vi "change_array_rows.vi"(9 "Scan Parameters 3":refnum<vi>, 10 "Scan Parameters":T1={"Initial Values"=[4.0], "Final Values"=[10.0, 0.0, 0.0], "Step Sizes"=[0.5, 0.0, 0.0], "Parameters to Change"=[enum."Static Voltage", enum."Static Voltage", enum."Static Voltage"], "Channels to Change"=[1.0, 0.0, 0.0], "Number of Parameters to Scan"=1, "Parameter Nickname (no spaces)"=["drop time"], "Scan Base Name"="BlueDetuning_", "Raw_Data Folder"=path "C:/Users/Rydberg/Documents/Data/Raw_Data/84Sr/2014.12.13"} {"Number of Parameters to Scan" min=1}) -> (2 "Scan Parameters 2":refnum<vi>)   [LabVIEW 2013]
uses:
  Controls/ScanParameters/ScanParametersPanel.ctl
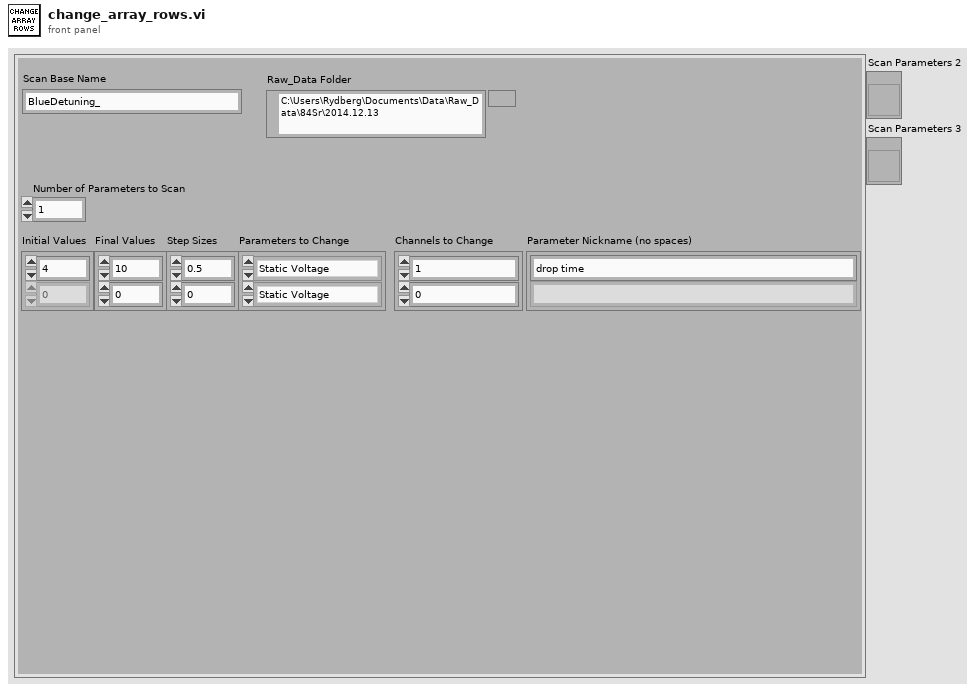
[diagram p1: front panel]
types:
  T1 = typedef "ScanParametersPanel.ctl" = cluster{"Initial Values":dbl[], "Final Values":dbl[], "Step Sizes":dbl[], "Parameters to Change":enum16{"PulseBlaster", "Static Voltage"}[], "Channels to Change":dbl[], "Number of Parameters to Scan":i32, "Parameter Nickname (no spaces)":string[], "Scan Base Name":string, "Raw_Data Folder":path}
  T2 = cluster{"Initial Values":refnum<vi>, "Final Values":refnum<vi>, "Step Sizes":refnum<vi>, "Channels to Change":refnum<vi>}
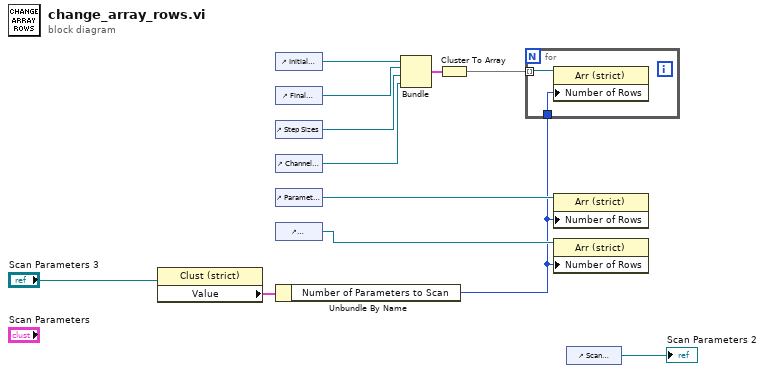
[diagram p0: block diagram]
diagram:
  n1 = property class="Clust (strict)"(reference="Scan Parameters 3") -> ("Value"=w1:T1)  [unwired: 1 in, 2 out]
  n2 = control-ref of="Initial Values"() -> (w11:refnum<vi>)
  n3 = control-ref of="Final Values"() -> (w10:refnum<vi>)
  n4 = control-ref of="Step Sizes"() -> (w9:refnum<vi>)
  n5 = control-ref of="Channels to Change"() -> (w8:refnum<vi>)
  n6 = control-ref of="Parameter Nickname (no spaces)"() -> (w6:refnum<vi>)
  n7 = control-ref of="Parameters to Change"() -> (w5:refnum<vi>)
  n8 = Unbundle By Name(w1) -> ("Number of Parameters to Scan"=w4:i32)
  n9 = Bundle("Initial Values"=w11, "Final Values"=w10, "Step Sizes"=w9, "Channels to Change"=w8) -> (w12:T2)  [unwired: 1 in]
  n10 = Cluster To Array(cluster=w12) -> (array=w7:refnum<vi>[])
  n11 = for {
    tunnel: w7 -> [w14] mode=indexing
    tunnel: w4 -> [w13]
    n12 = property class="Arr (strict)"(reference=w14, "Number of Rows"=w13) -> ()  [unwired: 1 in, 2 out]
  }
  n13 = property class="Arr (strict)"(reference=w6, "Number of Rows"=w4) -> ()  [unwired: 1 in, 2 out]
  n14 = property class="Arr (strict)"(reference=w5, "Number of Rows"=w4) -> ()  [unwired: 1 in, 2 out]
  n15 = control-ref of="Scan Parameters"() -> (→"Scan Parameters 2":refnum<vi>)
